vi "FGV Display.vi"(5 "FH 55 Gauss-/Teslameter":T1, 9 "action":enum16{"set", "get"}(ring)) -> (6 "FH 55 Gauss-/Teslameter 2":T1)   [LabVIEW 2014, in "FH 55.lvlib"]
doc: "In dieser FGV werden die Ausgabewerte des Displays gespeichert und ausgegeben. \n\nIn this FGV the output values are stored of the display."
uses:
  FH 55.lvlib
  TypeDef/Display.ctl
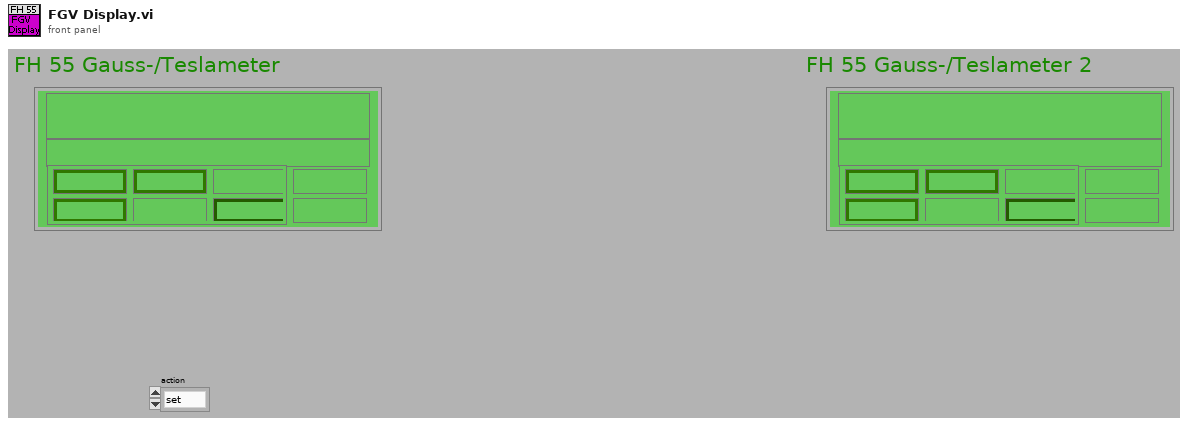
[diagram p1: front panel]
types:
  T1 = typedef "FH 55.lvlib/Display.ctl" = cluster{"current value":string, "Limit":string, "Remote":string, "function ":string, "Cluster":cluster{"AC/DC":string, "Auto":string, "Filter":string, "Range":string, "Rel":string, "Peak":string}}
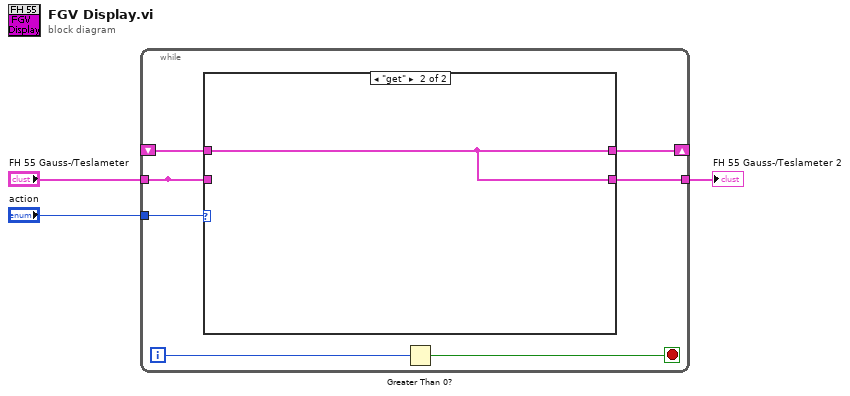
[diagram p0: block diagram]
diagram:
  n1 = while {
    tunnel: "FH 55 Gauss-/Teslameter" -> [w9]
    tunnel: [w9] -> _
    shift-right: [w7] -> _
    shift-left: _ -> [w10]
    tunnel: [w8] -> w1
    tunnel: "action" -> [w4]
    i -> [w6]
    stop <- w5 stop-if-true
    n2 = case shown="\"get\"" w4 {
      tunnel: w10 -> [_ w12]
      tunnel: w9 -> [w11 _]
      tunnel: [w11 w12] -> w8
      tunnel: [w11 w12] -> w7
      frame "set", Default {
      }
      frame "get" {
      }
    }
    n3 = Greater Than 0?(x=w6) -> (x > 0?=w5:bool)
  }
  "FH 55 Gauss-/Teslameter 2" <- w1
